vi "examen2.vi"() -> ()   [LabVIEW 2020]
uses:
  Control 1.ctl
panel:
  in  "Tab Control":enum32{"servicio", "mantenimiento"}(tab)
  in  "cancel":bool
  in  "COFFEE":bool
  in  "COLD DRINK":bool
  in  "CANDIES":bool
  in  "SNACKS":bool
  out "ESTADO":string
  out "dis 1":dbl
  out "dis 2":dbl
  out "dis 3":dbl
  out "dis 4":dbl
  in  "$20":bool
  in  "$10":bool
  out "$ INGRESADA":dbl
  out "$ DEVOLVER":dbl
  out "v. $10":dbl
  in  "RESET":bool
  in  "RESET SN":bool
  in  "RESET CO":bool
  in  "RESET CD":bool
  in  "RESET CA":bool
  out "v. $20":dbl
  # "MANTENIMIENTO"
  # "VALOR IN $ 10"
  # "VALOR IN $ 20"
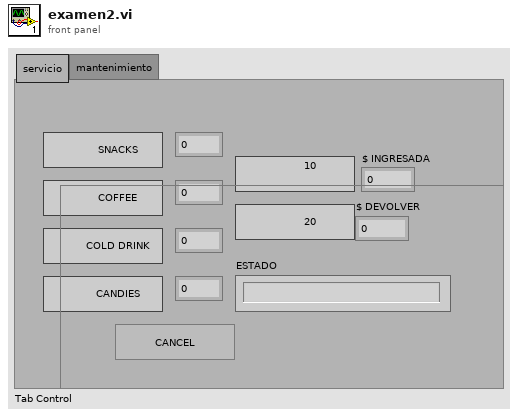
[diagram p1: front panel]
types:
  T1 = typedef "Control 1.ctl" = enum16{"inicio", "prod1", "prod2", "prod3", "prod4", "reset", "cancelar", "waiting1", "waiting2", "waiting3", "waiting4", "servi 1", "servi 2", "servi 3", "servi 4", "DIS1", "DIS2", "DIS3", "DIS4", "RETIRE PRODUCTO"}
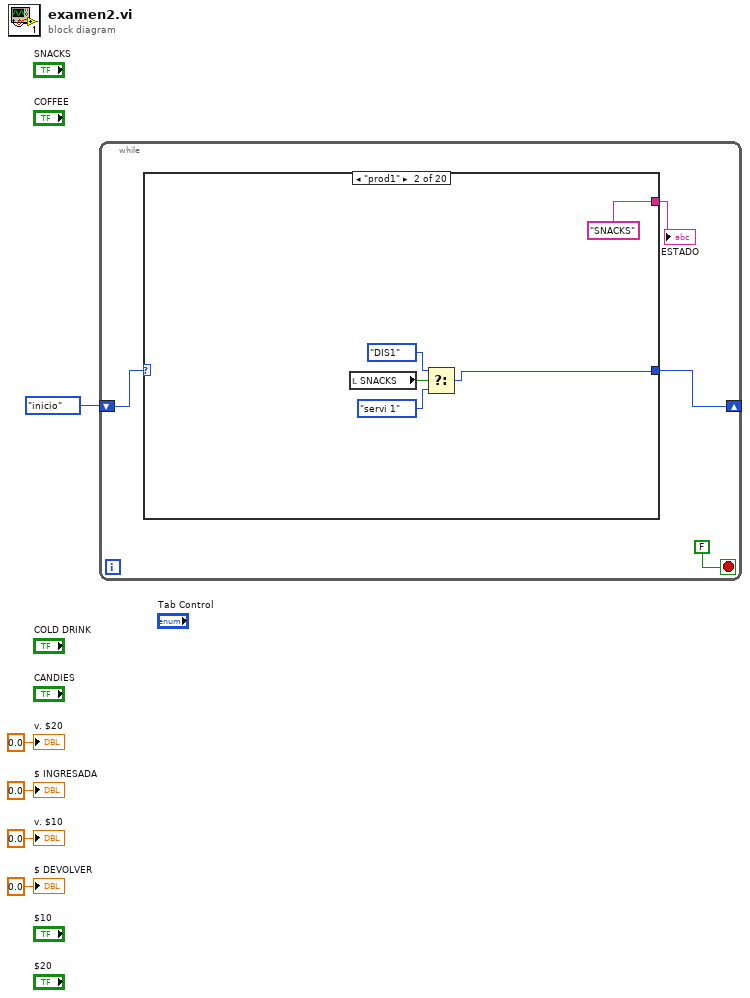
[diagram p0: block diagram]
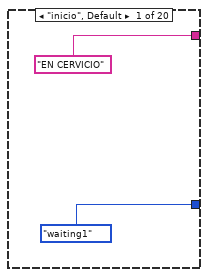
[diagram p2: hidden frame]
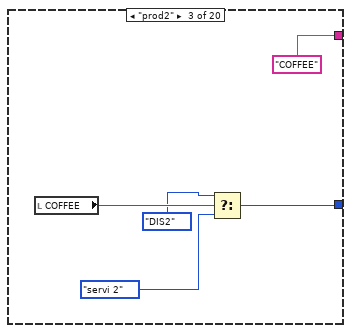
[diagram p3: hidden frame]
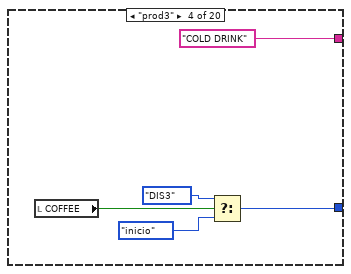
[diagram p4: hidden frame]
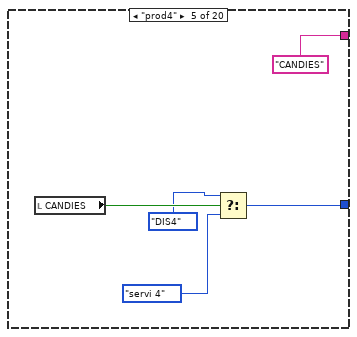
[diagram p5: hidden frame]
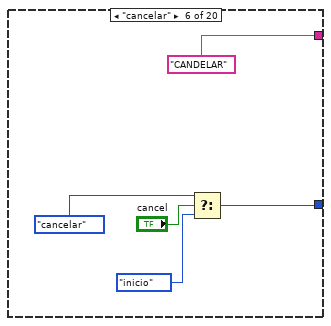
[diagram p6: hidden frame]
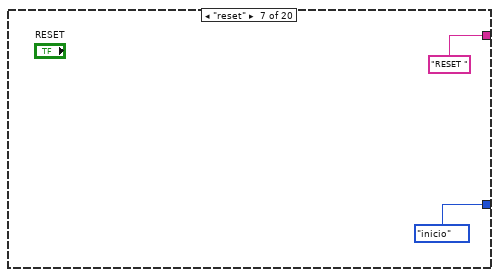
[diagram p7: hidden frame]
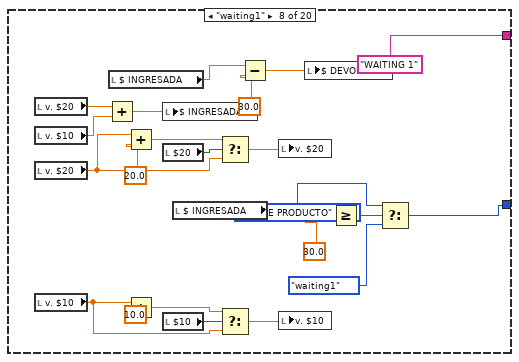
[diagram p8: hidden frame]
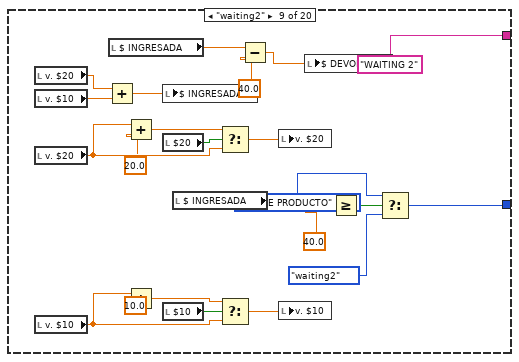
[diagram p9: hidden frame]
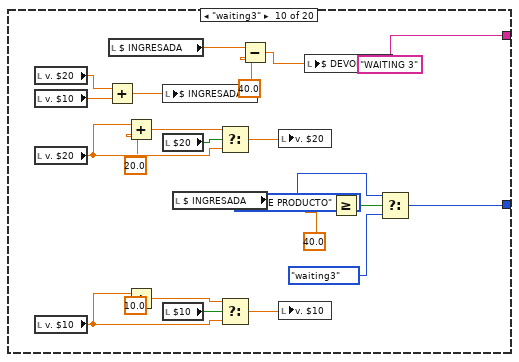
[diagram p10: hidden frame]
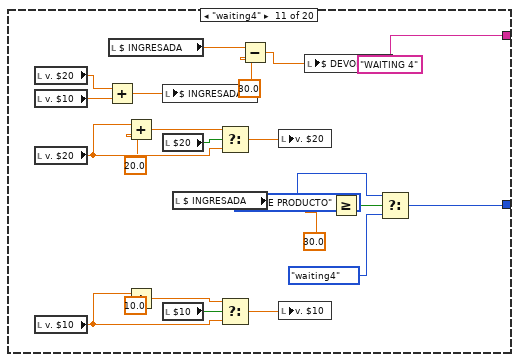
[diagram p11: hidden frame]
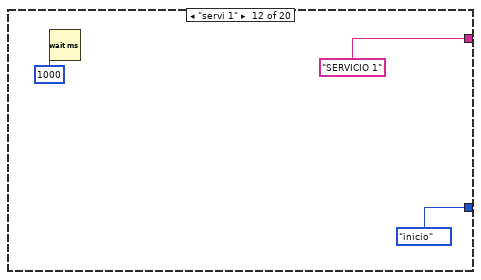
[diagram p12: hidden frame]
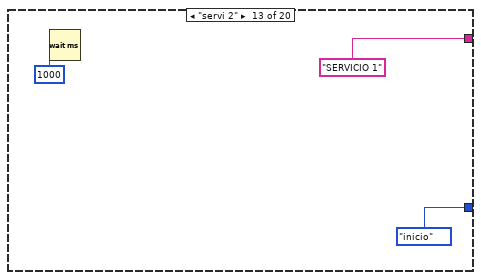
[diagram p13: hidden frame]
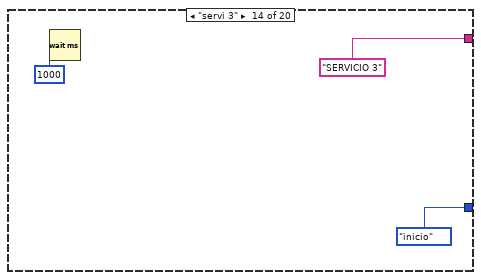
[diagram p14: hidden frame]
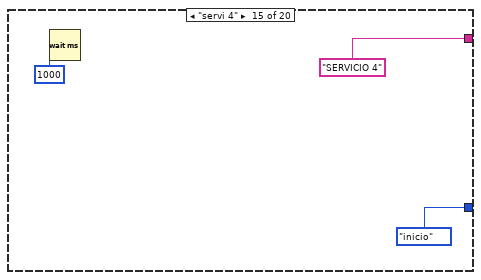
[diagram p15: hidden frame]
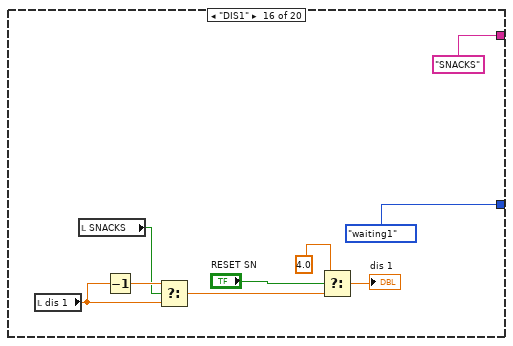
[diagram p16: hidden frame]
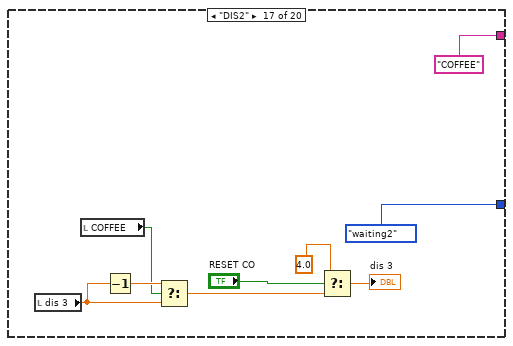
[diagram p17: hidden frame]
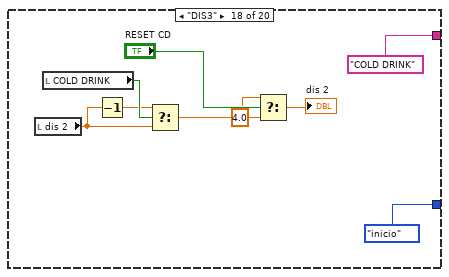
[diagram p18: hidden frame]
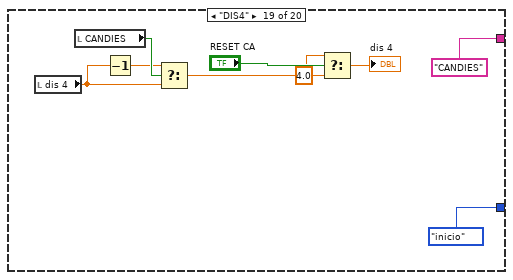
[diagram p19: hidden frame]
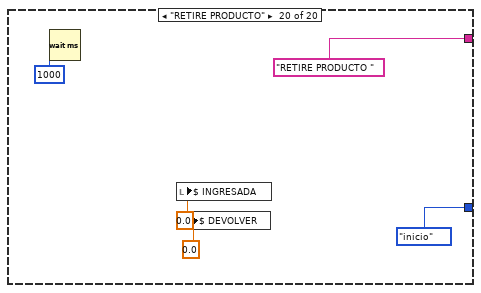
[diagram p20: hidden frame]
diagram:
  n1 = while {
    shift-right: [w7] -> _
    shift-left: Control_1."inicio" -> [w9]
    stop <- FALSE stop-if-true
    n2 = case shown="\"prod1\"" w9 {
      tunnel: [Control_1."waiting1" w12 w18 w23 w28 w33 Control_1."inicio" w39 w63 w86 w109 Control_1."inicio" Control_1."inicio" Control_1."inicio" Control_1."inicio" Control_1."waiting1" Control_1."waiting2" Control_1."inicio" Control_1."inicio" Control_1."inicio"] -> w7
      tunnel: ["EN CERVICIO" ("ESTADO") "SNACKS" ("ESTADO") "COFFEE" ("ESTADO") "COLD DRINK" ("ESTADO") "CANDIES" ("ESTADO") "CANDELAR" ("ESTADO") "RESET " ("ESTADO") "WAITING 1" ("ESTADO") "WAITING 2" ("ESTADO") "WAITING 3" ("ESTADO") "WAITING 4" ("ESTADO") "SERVICIO 1" ("ESTADO") "SERVICIO 1" ("ESTADO") "SERVICIO 3" ("ESTADO") "SERVICIO 4" ("ESTADO") "SNACKS" ("ESTADO") "COFFEE" ("ESTADO") "COLD DRINK" ("ESTADO") "CANDIES" ("ESTADO") "RETIRE PRODUCTO " ("ESTADO")] -> w6
      frame "inicio", Default {
      }
      frame "prod1" {
        n3 = local read "SNACKS"() -> (w15:bool)
        n4 = Select(t=Control_1."DIS1", s=w15, f=Control_1."servi 1") -> (s? t:f=w12:T1)
      }
      frame "prod2" {
        n5 = local read "COFFEE"() -> (w21:bool)
        n6 = Select(t=Control_1."DIS2", s=w21, f=Control_1."servi 2") -> (s? t:f=w18:T1)
      }
      frame "prod3" {
        n7 = local read "COFFEE"() -> (w26:bool)
        n8 = Select(t=Control_1."DIS3", s=w26, f=Control_1."inicio") -> (s? t:f=w23:T1)
      }
      frame "prod4" {
        n9 = local read "CANDIES"() -> (w31:bool)
        n10 = Select(t=Control_1."DIS4", s=w31, f=Control_1."servi 4") -> (s? t:f=w28:T1)
      }
      frame "cancelar" {
        n11 = Select(t=Control_1."cancelar", s="cancel", f=Control_1."inicio") -> (s? t:f=w33:T1)
      }
      frame "reset" {
      }
      frame "waiting1" {
        n12 = local read "v. $20"() -> (w60:dbl)
        n13 = local read "v. $10"() -> (w59:dbl)
        n14 = local read "v. $20"() -> (w56:dbl)
        n15 = local read "v. $10"() -> (w57:dbl)
        n16 = Add(x=w60, y=w59) -> (x+y=w50:dbl)
        n17 = local read "$ INGRESADA"() -> (w61:dbl)
        n18 = Add(x=w56, y=20.0) -> (x+y=w55:dbl)
        n19 = Add(x=w57, y=10.0) -> (x+y=w58:dbl)
        n20 = local write "$ INGRESADA"(w50) -> ()
        n21 = local read "$20"() -> (w46:bool)
        n22 = local read "$10"() -> (w47:bool)
        n23 = local read "$ INGRESADA"() -> (w45:dbl)
        n24 = Select(t=w55, s=w46, f=w56) -> (s? t:f=w51:dbl)
        n25 = Select(t=w58, s=w47, f=w57) -> (s? t:f=w49:dbl)
        n26 = Subtract(x=w61, y=30.0) -> (x-y=w48:dbl)
        n27 = local write "v. $20"(w51) -> ()
        n28 = local write "v. $10"(w49) -> ()
        n29 = local write "$ DEVOLVER"(w48) -> ()
        n30 = Greater Or Equal?(x=w45, y=30.0) -> (x >= y?=w43:bool)
        n31 = Select(t=Control_1."RETIRE PRODUCTO", s=w43, f=Control_1."waiting1") -> (s? t:f=w39:T1)
      }
      frame "waiting2" {
        n32 = local read "v. $20"() -> (w82:dbl)
        n33 = local read "v. $10"() -> (w81:dbl)
        n34 = local read "v. $20"() -> (w79:dbl)
        n35 = local read "v. $10"() -> (w62:dbl)
        n36 = Add(x=w82, y=w81) -> (x+y=w76:dbl)
        n37 = local read "$ INGRESADA"() -> (w83:dbl)
        n38 = Add(x=w79, y=20.0) -> (x+y=w78:dbl)
        n39 = Add(x=w62, y=10.0) -> (x+y=w80:dbl)
        n40 = local write "$ INGRESADA"(w76) -> ()
        n41 = local read "$20"() -> (w72:bool)
        n42 = local read "$10"() -> (w73:bool)
        n43 = local read "$ INGRESADA"() -> (w68:dbl)
        n44 = Select(t=w78, s=w72, f=w79) -> (s? t:f=w77:dbl)
        n45 = Select(t=w80, s=w73, f=w62) -> (s? t:f=w75:dbl)
        n46 = Subtract(x=w83, y=40.0) -> (x-y=w74:dbl)
        n47 = local write "v. $20"(w77) -> ()
        n48 = local write "v. $10"(w75) -> ()
        n49 = local write "$ DEVOLVER"(w74) -> ()
        n50 = Greater Or Equal?(x=w68, y=40.0) -> (x >= y?=w66:bool)
        n51 = Select(t=Control_1."RETIRE PRODUCTO", s=w66, f=Control_1."waiting2") -> (s? t:f=w63:T1)
      }
      frame "waiting3" {
        n52 = local read "v. $20"() -> (w105:dbl)
        n53 = local read "v. $10"() -> (w104:dbl)
        n54 = local read "v. $20"() -> (w102:dbl)
        n55 = local read "v. $10"() -> (w85:dbl)
        n56 = Add(x=w105, y=w104) -> (x+y=w99:dbl)
        n57 = local read "$ INGRESADA"() -> (w106:dbl)
        n58 = Add(x=w102, y=20.0) -> (x+y=w101:dbl)
        n59 = Add(x=w85, y=10.0) -> (x+y=w103:dbl)
        n60 = local write "$ INGRESADA"(w99) -> ()
        n61 = local read "$20"() -> (w95:bool)
        n62 = local read "$10"() -> (w96:bool)
        n63 = local read "$ INGRESADA"() -> (w91:dbl)
        n64 = Select(t=w101, s=w95, f=w102) -> (s? t:f=w100:dbl)
        n65 = Select(t=w103, s=w96, f=w85) -> (s? t:f=w98:dbl)
        n66 = Subtract(x=w106, y=40.0) -> (x-y=w97:dbl)
        n67 = local write "v. $20"(w100) -> ()
        n68 = local write "v. $10"(w98) -> ()
        n69 = local write "$ DEVOLVER"(w97) -> ()
        n70 = Greater Or Equal?(x=w91, y=40.0) -> (x >= y?=w90:bool)
        n71 = Select(t=Control_1."RETIRE PRODUCTO", s=w90, f=Control_1."waiting3") -> (s? t:f=w86:T1)
      }
      frame "waiting4" {
        n72 = local read "v. $20"() -> (w128:dbl)
        n73 = local read "v. $10"() -> (w127:dbl)
        n74 = local read "v. $20"() -> (w125:dbl)
        n75 = local read "v. $10"() -> (w108:dbl)
        n76 = Add(x=w128, y=w127) -> (x+y=w122:dbl)
        n77 = local read "$ INGRESADA"() -> (w129:dbl)
        n78 = Add(x=w125, y=20.0) -> (x+y=w124:dbl)
        n79 = Add(x=w108, y=10.0) -> (x+y=w126:dbl)
        n80 = local write "$ INGRESADA"(w122) -> ()
        n81 = local read "$20"() -> (w118:bool)
        n82 = local read "$10"() -> (w119:bool)
        n83 = local read "$ INGRESADA"() -> (w114:dbl)
        n84 = Select(t=w124, s=w118, f=w125) -> (s? t:f=w123:dbl)
        n85 = Select(t=w126, s=w119, f=w108) -> (s? t:f=w121:dbl)
        n86 = Subtract(x=w129, y=30.0) -> (x-y=w120:dbl)
        n87 = local write "v. $20"(w123) -> ()
        n88 = local write "v. $10"(w121) -> ()
        n89 = local write "$ DEVOLVER"(w120) -> ()
        n90 = Greater Or Equal?(x=w114, y=30.0) -> (x >= y?=w112:bool)
        n91 = Select(t=Control_1."RETIRE PRODUCTO", s=w112, f=Control_1."waiting4") -> (s? t:f=w109:T1)
      }
      frame "servi 1" {
        n92 = Wait (ms)(milliseconds to wait=u32 1000) -> ()  [unwired: 1 out]
      }
      frame "servi 2" {
        n93 = Wait (ms)(milliseconds to wait=u32 1000) -> ()  [unwired: 1 out]
      }
      frame "servi 3" {
        n94 = Wait (ms)(milliseconds to wait=u32 1000) -> ()  [unwired: 1 out]
      }
      frame "servi 4" {
        n95 = Wait (ms)(milliseconds to wait=u32 1000) -> ()  [unwired: 1 out]
      }
      frame "DIS1" {
        n96 = local read "dis 1"() -> (w146:dbl)
        n97 = local read "SNACKS"() -> (w148:bool)
        n98 = Decrement(x=w146) -> (x-1=w150:dbl)
        n99 = Select(t=w150, s=w148, f=w146) -> (s? t:f=w151:dbl)
        n100 = Select(t=4.0, s="RESET SN", f=w151) -> (s? t:f=→"dis 1":dbl)
      }
      frame "DIS2" {
        n101 = local read "dis 3"() -> (w157:dbl)
        n102 = local read "COFFEE"() -> (w155:bool)
        n103 = Decrement(x=w157) -> (x-1=w158:dbl)
        n104 = Select(t=w158, s=w155, f=w157) -> (s? t:f=w159:dbl)
        n105 = Select(t=4.0, s="RESET CO", f=w159) -> (s? t:f=→"dis 3":dbl)
      }
      frame "DIS3" {
        n106 = local read "dis 2"() -> (w166:dbl)
        n107 = local read "COLD DRINK"() -> (w168:bool)
        n108 = Decrement(x=w166) -> (x-1=w165:dbl)
        n109 = Select(t=w165, s=w168, f=w166) -> (s? t:f=w164:dbl)
        n110 = Select(t=4.0, s="RESET CD", f=w164) -> (s? t:f=→"dis 2":dbl)
      }
      frame "DIS4" {
        n111 = local read "dis 4"() -> (w175:dbl)
        n112 = local read "CANDIES"() -> (w177:bool)
        n113 = Decrement(x=w175) -> (x-1=w174:dbl)
        n114 = Select(t=w174, s=w177, f=w175) -> (s? t:f=w173:dbl)
        n115 = Select(t=4.0, s="RESET CA", f=w173) -> (s? t:f=→"dis 4":dbl)
      }
      frame "RETIRE PRODUCTO" {
        n116 = Wait (ms)(milliseconds to wait=u32 1000) -> ()  [unwired: 1 out]
        n117 = local write "$ INGRESADA"(0.0 ("$ INGRESADA")) -> ()
        n118 = local write "$ DEVOLVER"(0.0 ("$ DEVOLVER")) -> ()
      }
    }
    "ESTADO" <- w6
  }
  "v. $20" <- 0.0 ("v. $20")
  "$ INGRESADA" <- 0.0 ("$ INGRESADA")
  "v. $10" <- 0.0 ("v. $10")
  "$ DEVOLVER" <- 0.0 ("$ DEVOLVER")
